vi "Parabolic Cylinder Function.vi"(2 "v":dbl format="%.2f", 3 "x":dbl format="%.2f") -> (1 "Dv(x)":dbl format="%.2f")   [LabVIEW 2020, in "NI_Gmath.lvlib"]
doc: "Computes the parabolic cylinder, or Weber, function."
uses:
  NI_Gmath.lvlib
  <resource>/lvanlys.dll
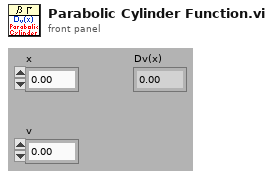
[diagram p1: front panel]
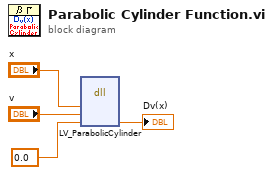
[diagram p0: block diagram]
diagram:
  n1 = dll-call lib="C:/Program Files (x86)/National Instruments/LabVIEW 2020/resource/lvanlys.*" fn="LV_ParabolicCylinder"("x"="x", "v"="v", "Dv(x)"=0.0 ("cylinder")) -> ("Dv(x)"=→"Dv(x)":dbl)  [unwired: 6 in, 2 out]
